vi "Read Write AVI With Data.vi"() -> ()   [LabVIEW 2014]
doc: "Demonstrates how to use the Legacy AVI functions to create and read an AVI with custom data associated with each frame. The Legacy VIs are used because the current VIs do not currently support data associated with each frame."
panel:
  out "Image":T1(plugin-control)
  out "Data":T2
  in  "Frame and Data to Examine":i32(slide) max=165 scale=0.0..165.0
  in  "Stop":bool
  # "Overview: Demonstrates how to use the Legacy AVI functions to create and read an AVI with custom data associated with each frame. The Legacy VIs are used because the current VIs do not currently support data associated with each frame.\nRequirements: Vision Development Software.\nInstructions:\n1. Run the VI.\n2. Change the Frame and Data to Examine to see the image and corresponding data that was saved to the AVI."
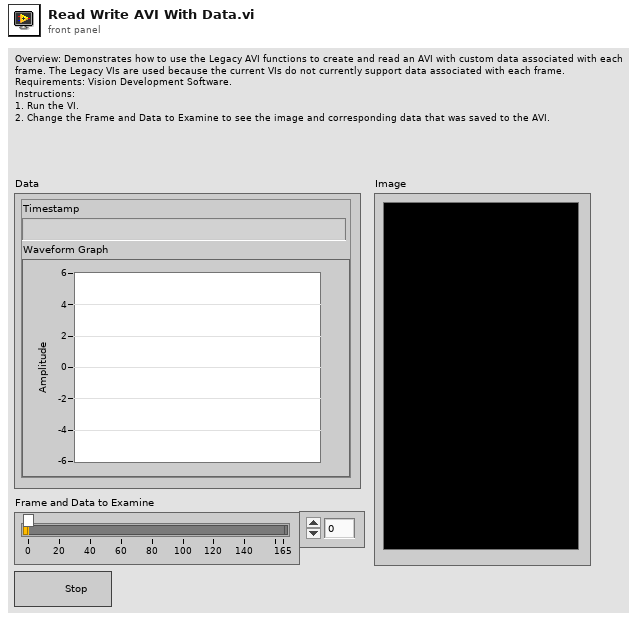
[diagram p1: front panel]
types:
  T1 = typedef "IMAQ Image.ctl" = refnum<image>
  T2 = cluster{"Timestamp":string, "Waveform Graph":waveform(dbl)[]}
  T3 = enum8{"Enabled", "Disabled", "Disabled and Grayed Out"}
  T4 = typedef "AviRefnum.ctl" = refnum<k1>
  T5 = cluster{"date/time string":string, "Simulated Waveform Data":waveform(dbl)[]}
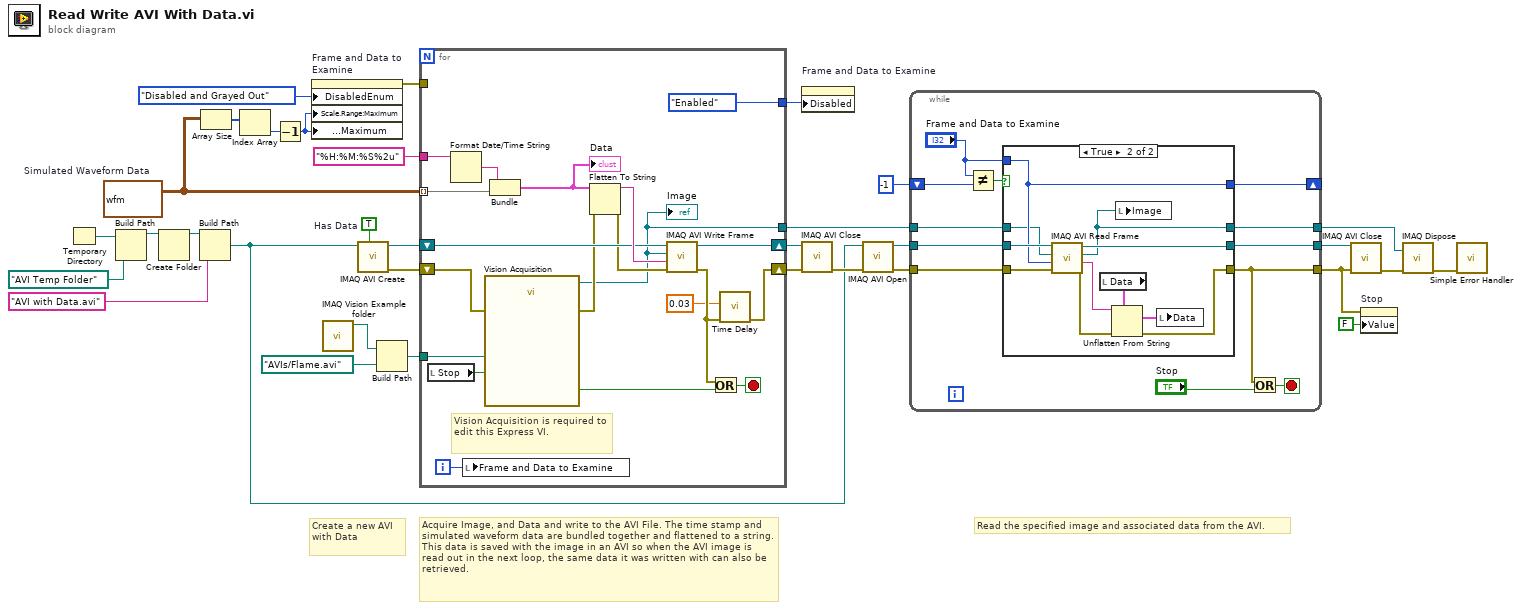
[diagram p0: block diagram]
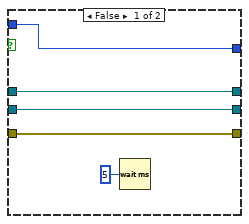
[diagram p2: hidden frame]
diagram:
  w9 = waveform(dbl)[][] data[426794B]  # Simulated Waveform Data
  w28 = TRUE  # Has Data
  # "Read the specified image and associated data from the AVI."
  # "Create a new AVI with Data"
  # "Acquire Image, and Data and write to the AVI File. The time stamp and simulated waveform data are bundled together and flattened to a string.  This data is saved with the image in an AVI so when the AVI image is read out in the next loop, the same data it was written with can also be retrieved."
  n1 = Temporary Directory() -> (w2:path)
  n2 = Build Path(base path=w2, name or relative path=path "AVI Temp Folder") -> (appended path=w23:path)
  n3 = Create Folder(path (use dialog)=w23) -> (created path=w22:path)  [unwired: 1 in, 3 out]
  n4 = Build Path(base path=w22, name or relative path="AVI with Data.avi") -> (appended path=w13:path)
  n5 = Array Size(array=w9) -> (size(s)=w8:i32[])
  n6 = Index Array(array=w8) -> (element=w7:i32)  [unwired: 1 in]
  n7 = Decrement(x=w7) -> (x-1=w3:i32)
  n8 = property on="Frame and Data to Examine" class="Slide (strict)"("DisabledEnum"=T3."Disabled and Grayed Out" ("Disabled"), "Scale.Range:Maximum"=w3, "Data Entry Limits:Maximum"=w3) -> (error out=w11:errorcluster)  [unwired: 2 in, 1 out]
  n9 = call "IMAQ Vision Example folder.vi"() -> ("Example Image Path"=w27:path)  [unwired: 11 in]
  n10 = call "IMAQ AVI Create"("Has Data"=w28, "AVI Path"=w13) -> ("error out"=w18:errorcluster, "Avi Refnum"=w19:T4)  [unwired: 8 in]
  n11 = Build Path(base path=w27, name or relative path=path "AVIs/Flame.avi") -> (appended path=w25:path)
  n12 = for {
    tunnel: w25 -> [w53]
    tunnel: w9 -> [w36] mode=indexing
    tunnel: "%H:%M:%S%2u" ("time format string (%c)") -> [w50]
    shift-right: [w47] -> w16
    shift-left: w19 -> [w44]
    shift-right: [w34] -> w17
    shift-left: w18 -> [w49]
    tunnel: [w38] -> w1
    tunnel: [T3."Enabled" ("Disabled")] -> w12
    tunnel: w11 -> [_]
    i -> [w37]
    stop <- w45 stop-if-true
    # "Vision Acquisition is required to edit this Express VI."
    n13 = local read "Stop"() -> (w52:bool)
    n14 = Format Date/Time String(time format string (%c)=w50) -> (date/time string=w51:string)  [unwired: 2 in]
    n15 = local write "Frame and Data to Examine"(w37) -> ()
    n16 = call "Vision Acquisition"("AVI Path"=w53, "Stop (F)"=w52, "error in"=w49) -> ("Image Out"=w38:T1, "Stopped"=w46:bool, "error out"=w43:errorcluster)  [unwired: 22 in]
    "Image" <- w38
    n17 = Bundle("date/time string"=w51, "Simulated Waveform Data"=w36) -> (w35:T5)  [unwired: 1 in]
    "Data" <- w35
    n18 = Flatten To String(anything=w35, error in (no error)=w43) -> (data string=w48:string, error out=w42:errorcluster)  [unwired: 2 in, 1 out]
    n19 = call "IMAQ AVI Write Frame"("error in (no error)"=w42, "Data"=w48, "Image"=w38, "Avi Refnum"=w44) -> ("error out"=w41:errorcluster, "Avi Refnum (duplicate)"=w47:T4)  [unwired: 6 in]
    n20 = Or(x=w41, y=w46) -> (x .or. y?=w45:bool)
    n21 = call "Time Delay"("error in (no error)"=w41, "Delay Time (s)"=0.03) -> ("error out"=w34:errorcluster)  [unwired: 9 in]
  }
  n22 = property on="Frame and Data to Examine" class="Slide (strict)"("Disabled"=w12) -> ()  [unwired: 2 in, 2 out]
  n23 = call "IMAQ AVI Close"("error in (no error)"=w17, "Avi Refnum"=w16) -> ("error out"=w14:errorcluster)  [unwired: 9 in]
  n24 = call "IMAQ AVI Open"("error in (no error)"=w14, "AVI Path"=w13) -> ("error out"=w15:errorcluster, "Avi Refnum"=w31:T4)  [unwired: 8 in]
  n25 = while {
    tunnel: [w58] -> w32
    tunnel: [w55] -> w6
    tunnel: [w61] -> w29
    shift-left: -1 -> [w65]
    shift-right: [w59] -> _
    tunnel: w31 -> [w63]
    tunnel: w15 -> [w62]
    tunnel: w1 -> [w57]
    stop <- w54 stop-if-true
    n26 = Not Equal?(x="Frame and Data to Examine", y=w65) -> (x != y?=w64:bool)
    n27 = case shown="True" w64 {
      tunnel: w63 -> [w69 w81]
      tunnel: w62 -> [w68 w80]
      tunnel: "Frame and Data to Examine" -> [w67 w77]
      tunnel: [w69 w78] -> w61
      tunnel: [w68 w73] -> w55
      tunnel: [w67 w77] -> w59
      tunnel: [w66 w75] -> w58
      tunnel: w57 -> [w66 w76]
      frame False {
        n28 = Wait (ms)(milliseconds to wait=u32 5) -> ()  [unwired: 1 out]
      }
      frame True {
        n29 = call "IMAQ AVI Read Frame"("error in (no error)"=w80, "Frame Number"=w77, "Image"=w76, "Avi Refnum"=w81) -> ("error out"=w74:errorcluster, "Data Out"=w79:string, "Image Out"=w75:T1, "Avi Refnum (duplicate)"=w78:T4)  [unwired: 4 in]
        n30 = local read "Data"() -> (w71:T2)
        n31 = Unflatten From String(type=w71, binary string=w79, error in (no error)=w74) -> (value=w72:T2, error out=w73:errorcluster)  [unwired: 2 in, 1 out]
        n32 = local write "Image"(w75) -> ()
        n33 = local write "Data"(w72) -> ()
      }
    }
    n34 = Or(x=w55, y="Stop") -> (x .or. y?=w54:bool)
  }
  n35 = call "IMAQ AVI Close"("error in (no error)"=w6, "Avi Refnum"=w29) -> ("error out"=w33:errorcluster)  [unwired: 9 in]
  n36 = property on="Stop" class="Bool (strict)"(error in=w6, "Value"=FALSE ("Stop")) -> ()  [unwired: 1 in, 2 out]
  n37 = call "IMAQ Dispose"("Image"=w32, "error in (no error)"=w33) -> ("error out"=w4:errorcluster)  [unwired: 4 in]
  n38 = call <vilib>:"Simple Error Handler.vi"("error in (no error)"=w4) -> ()  [unwired: 4 in, 5 out]
